vi "Get PPL Version Application.vi"() -> ()   [LabVIEW 2019]
uses:
  <vilib>/Wiresmith Technology/G CLI/CLI Class/CLI.lvclass
  <vilib>/Utility/LVLibp/NI_PackedLibraryUtility.lvlib
panel:
  in  "packed library path":path
  out "Version":string
  out "Commit Reference":string
  out "error out":errorcluster
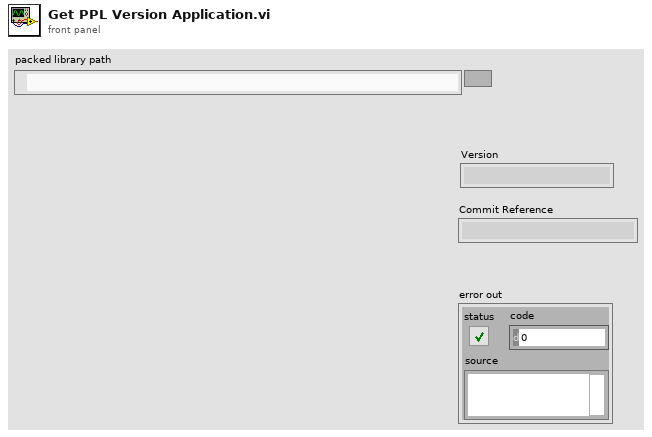
[diagram p1: front panel]
types:
  T1 = enum32{"Invalid", "Standard", "Closed", "Hidden", "Minimized", "Maximized"}
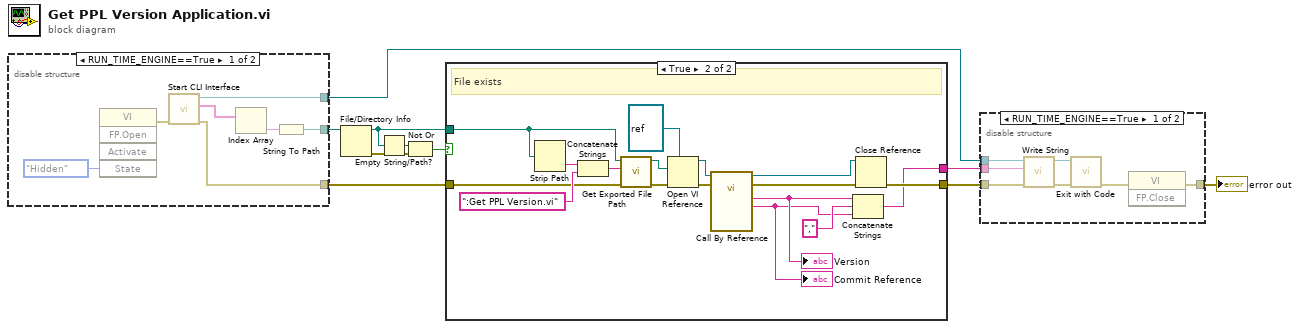
[diagram p0: block diagram]
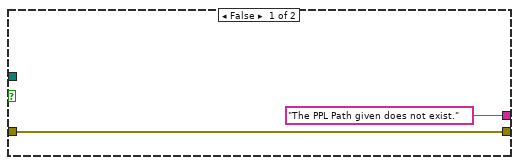
[diagram p2: hidden frame]
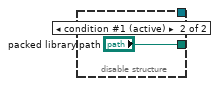
[diagram p3: hidden frame]
diagram:
  n1 = disable-structure shown="RUN_TIME_ENGINE==True" {
    disable-tunnel: [w16 "packed library path"] -> w10
    disable-tunnel: [w15 _] -> w7
    disable-tunnel: [w14 _] -> w6
    frame condition #0 {
      n2 = invoke class="VI" method="FP.Open"("State"=T1."Hidden") -> (error out=w11:errorcluster)  [unwired: 4 in, 4 out]
      n3 = call <vilib>:"Start CLI Interface.vi"("error in (no error)"=w11) -> ("error out"=w14:errorcluster, "Custom Parameters"=w12:string[], "CLI out"=w15:refnum<class "CLI.lvclass">)  [unwired: 8 in]
      n4 = Index Array(array=w12) -> (element=w13:string)  [unwired: 1 in]
      n5 = String To Path(string=w13) -> (path=w16:path)
    }
    frame condition #1 (active) {
    }
  }
  n6 = File/Directory Info(path=w10) -> (path out=w4:path, error out=w2:errorcluster)  [unwired: 1 in, 5 out]
  n7 = Empty String/Path?(string/path=w4) -> (empty?=w3:bool)
  n8 = Not Or(1:w2, 2:w3) -> (0:w1:bool)
  n9 = case shown="True" w1 {
    tunnel: [w20 w27] -> w9
    tunnel: w6 -> [w20 w26]
    tunnel: ["The PPL Path given does not exist." w23] -> w5
    tunnel: w4 -> [_ w21]
    frame False {
    }
    frame True {
      # "File exists"
      n10 = Strip Path(path=w21) -> (name=w30:string)  [unwired: 1 out]
      n11 = Concatenate Strings(w30, ":Get PPL Version.vi" ("string")) -> (w28:string)
      n12 = call <vilib>:"Get Exported File Path.vi"("error in (no error)"=w26, "qualified name"=w28, "packed library path"=w21) -> ("error out"=w35:errorcluster, "path"=w37:path)  [unwired: 7 in]
      n13 = Open VI Reference(type specifier VI Refnum (for type only)=refnum<vi> refnum, vi path=w37, error in (no error)=w35) -> (vi reference=w32:refnum<vi>, error out=w36:errorcluster)  [unwired: 3 in]
      n14 = call-by-ref "?"(reference=w32, error in=w36) -> (reference out=w33:refnum<vi>, error out=w34:errorcluster, "Commit Reference"=w22:string, "Version"=w25:string)  [unwired: 10 in]
      "Commit Reference" <- w22
      "Version" <- w25
      n15 = Concatenate Strings(w25, "," ("string"), w22) -> (w23:string)
      n16 = Close Reference(reference=w33, error in (no error)=w34) -> (error out=w27:errorcluster)
    }
  }
  n17 = disable-structure shown="RUN_TIME_ENGINE==True" {
    disable-tunnel: w9 -> [w42 w45]
    disable-tunnel: [w44 w45] -> w8
    disable-tunnel: w7 -> [w43 _]
    disable-tunnel: w5 -> [w38 _]
    frame condition #0 {
      n18 = call <vilib>:"Write String.vi"("error in (no error)"=w42, "Text to Write"=w38, "CLI in"=w43) -> ("error out"=w39:errorcluster, "CLI out"=w40:refnum<class "CLI.lvclass">)  [unwired: 7 in]
      n19 = call <vilib>:"Exit with Code.vi"("error in (no error)"=w39, "CLI in"=w40) -> ("error out"=w41:errorcluster)  [unwired: 9 in]
      n20 = invoke class="VI" method="FP.Close"(error in=w41) -> (error out=w44:errorcluster)  [unwired: 2 in, 2 out]
    }
    frame condition #1 (active) {
    }
  }
  "error out" <- w8
